vi "CRYSelect Graph Window by Tab.vi"(10 "pGraph VIs In":refnum<vi>[](array[refnum]), 11 "Type":enum16{"Curves", "Values", "Results", "WFM"}(ring)) -> (3 "pGraph VIs Out":refnum<vi>[](array[refnum]))   [LabVIEW 2013]
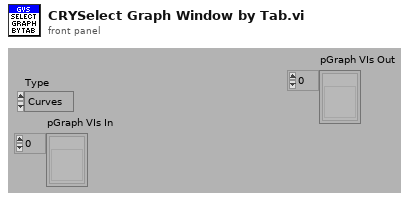
[diagram p1: front panel]
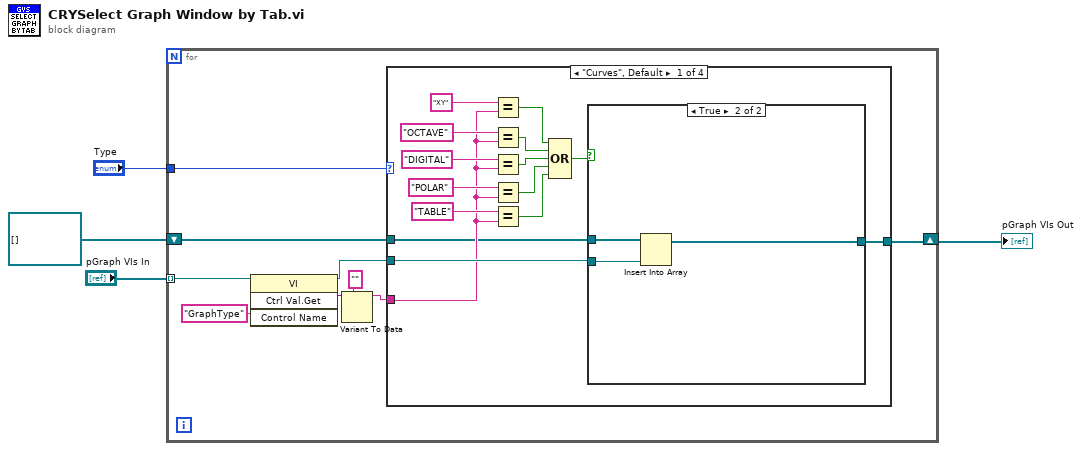
[diagram p0: block diagram]
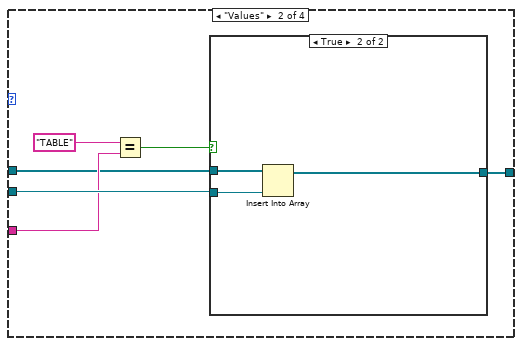
[diagram p3: hidden frame]
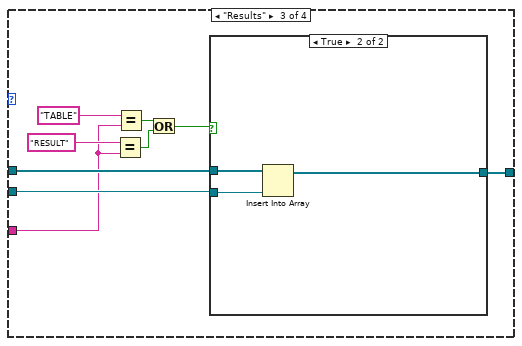
[diagram p5: hidden frame]
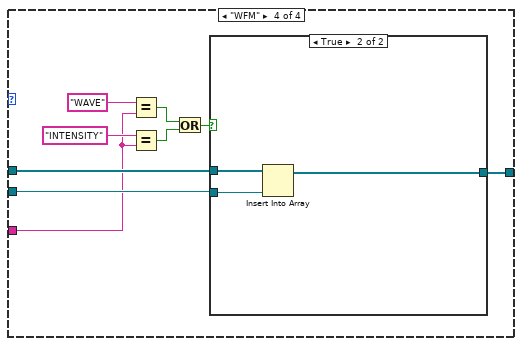
[diagram p7: hidden frame]
diagram:
  n1 = for {
    tunnel: "Type" -> [w11]
    tunnel: "pGraph VIs In" -> [w7] mode=indexing
    shift-right: [w12] -> w3
    shift-left: refnum<vi>[] [] ("Graph VI Ref") -> [w13]
    n2 = invoke class="VI" method="Ctrl Val.Get"(reference=w7, "Control Name"="GraphType") -> (reference out=w5:refnum<vi>, "Get Control Value Variant"=w8:variant)  [unwired: 2 in, 2 out]
    n3 = Variant To Data(type="", Variant=w8) -> (data=w6:string)  [unwired: 1 in, 1 out]
    n4 = case shown="\"Curves\", Default" w11 {
      tunnel: w6 -> [w17 w36 w46 w56]
      tunnel: w5 -> [w28 w38 w51 w64]
      tunnel: w13 -> [w15 w35 w49 w62]
      tunnel: [w14 w34 w48 w61] -> w12
      frame "Curves", Default {
        n5 = Equal?(x="XY", y=w17) -> (x = y?=w23:bool)
        n6 = Equal?(x="OCTAVE", y=w17) -> (x = y?=w22:bool)
        n7 = Equal?(x="DIGITAL", y=w17) -> (x = y?=w21:bool)
        n8 = Equal?(x="POLAR", y=w17) -> (x = y?=w20:bool)
        n9 = Equal?(x="TABLE", y=w17) -> (x = y?=w16:bool)
        n10 = Compound Arithmetic op=OR(w23, w22, w21, w20, w16) -> (w19:bool)
        n11 = case shown="True" w19 {
          tunnel: w28 -> [_ w31]
          tunnel: w15 -> [w29 w32]
          tunnel: [w29 w30] -> w14
          frame False {
          }
          frame True {
            n12 = Insert Into Array(array=w32, new element=w31) -> (w30:refnum<vi>[])  [unwired: 1 in]
          }
        }
      }
      frame "Values" {
        n13 = Equal?(x="TABLE", y=w36) -> (x = y?=w33:bool)
        n14 = case shown="True" w33 {
          tunnel: w38 -> [_ w41]
          tunnel: w35 -> [w39 w42]
          tunnel: [w39 w40] -> w34
          frame False {
          }
          frame True {
            n15 = Insert Into Array(array=w42, new element=w41) -> (w40:refnum<vi>[])  [unwired: 1 in]
          }
        }
      }
      frame "Results" {
        n16 = Equal?(x="RESULT", y=w46) -> (x = y?=w44:bool)
        n17 = Equal?(x="TABLE", y=w46) -> (x = y?=w45:bool)
        n18 = Or(x=w45, y=w44) -> (x .or. y?=w43:bool)
        n19 = case shown="True" w43 {
          tunnel: w51 -> [_ w54]
          tunnel: w49 -> [w52 w55]
          tunnel: [w52 w53] -> w48
          frame False {
          }
          frame True {
            n20 = Insert Into Array(array=w55, new element=w54) -> (w53:refnum<vi>[])  [unwired: 1 in]
          }
        }
      }
      frame "WFM" {
        n21 = Equal?(x="WAVE", y=w56) -> (x = y?=w58:bool)
        n22 = Equal?(x="INTENSITY", y=w56) -> (x = y?=w59:bool)
        n23 = Or(x=w58, y=w59) -> (x .or. y?=w57:bool)
        n24 = case shown="True" w57 {
          tunnel: w64 -> [_ w67]
          tunnel: w62 -> [w65 w68]
          tunnel: [w65 w66] -> w61
          frame False {
          }
          frame True {
            n25 = Insert Into Array(array=w68, new element=w67) -> (w66:refnum<vi>[])  [unwired: 1 in]
          }
        }
      }
    }
  }
  "pGraph VIs Out" <- w3
